vi "SetSerial_Dialog.vi"(11 "error in (no error)":errorcluster) -> (6 "Cancelled?":bool=TRUE, 15 "error out":errorcluster)   [LabVIEW 2009]
doc: "Dialog box interface that lets user select serial port where scanner is located. If user hits OK, a connection to the specified port is attempted."
uses:
  globals/VISAResourceName.vi
panel:
  in  "OK":bool
  in  "Scanner Serial Port":refnum<visa-resource-name>="USB_Serial"
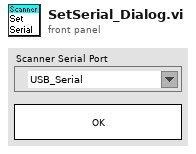
[diagram p1: front panel]
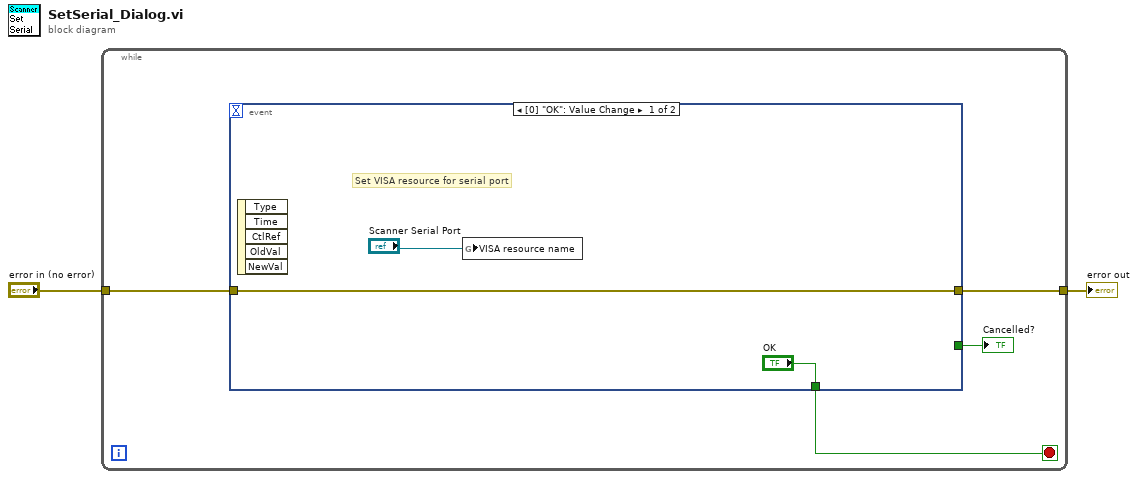
[diagram p0: block diagram]
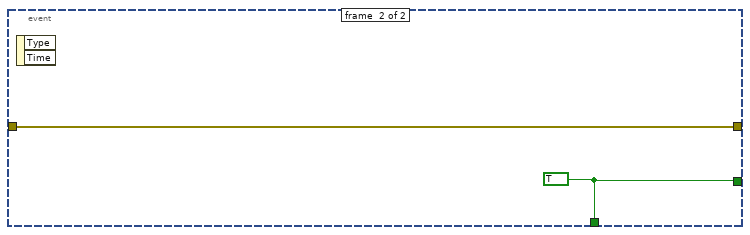
[diagram p2: hidden frame]
diagram:
  n1 = while {
    tunnel: [w5] -> w2
    tunnel: "error in (no error)" -> [w4]
    stop <- w6 stop-if-true
    n2 = event shown="[0] \"OK\": Value Change" {
      selector: _ -> [_ _]
      dyn-events: _ -> [_ _]
      timeout: _ -> [_ _]
      tunnel: ["OK" w10] -> w6
      tunnel: [w7 w11] -> w5
      tunnel: w4 -> [w7 w11]
      tunnel: [_ w10] -> w3
      event #0 {
        # "Set VISA resource for serial port"
        n3 = event-data() -> ()  [unwired: 1 in, 5 out]
        n4 = global write "VISAResourceName.vi" "VISA resource name"("Scanner Serial Port") -> ()
      }
      event #1 {
        w10 = TRUE
        n5 = event-data() -> ()  [unwired: 1 in, 2 out]
      }
    }
    "Cancelled?" <- w3
  }
  "error out" <- w2
